vi "SendCommand3.vi"(2 "timeout ms":i32=10000, 3 "command":string) -> (0 "reply":string="\r\n", 1 "Error":bool)   [LabVIEW 2014]
uses:
  EngineeringGlobals.vi
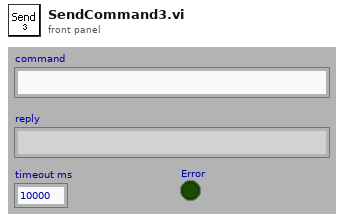
[diagram p1: front panel]
types:
  T1 = enum16{"Standard", "Buffered", "CRLF", "Immediate"}
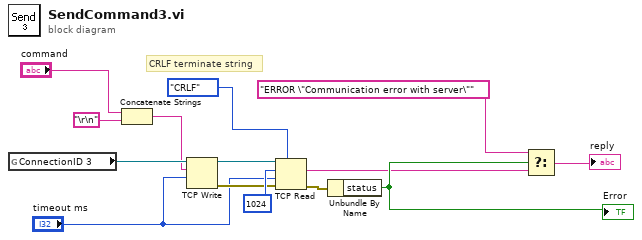
[diagram p0: block diagram]
diagram:
  # "CRLF terminate string"
  n1 = global read "EngineeringGlobals.vi" "ConnectionID 3"() -> (w6:refnum<k5>)
  n2 = Concatenate Strings("command", "\r\n") -> (w4:string)
  n3 = TCP Write(connection ID=w6, data in=w4, 9:"timeout ms") -> (connection ID out=w11:refnum<k5>, error out=w9:errorcluster)  [unwired: 1 in, 1 out]
  n4 = TCP Read(connection ID=w11, bytes to read=1024, error in (no error)=w9, 7:T1."CRLF" ("mode (standard)"), 9:"timeout ms") -> (data out=w3:string, error out=w2:errorcluster)  [unwired: 1 out]
  n5 = Unbundle By Name(w2) -> ("status"=w12:bool)
  "Error" <- w12
  n6 = Select(t="ERROR \"Communication error with server\"" ("data out"), s=w12, f=w3) -> (s? t:f=→"reply":string)
